vi "releaseQueue.vi"(8 "Error In":errorcluster, 11 "MissionQueue.lvclass":refnum<class "MissionQueue.lvclass">) -> (0 "Error Out":errorcluster, 2 "remaining elements":refnum<class "Mission.lvclass">[](array[class]))   [LabVIEW 2011, in "MissionQueue.lvclass"]
doc: "Close the MissionQueue reference and returning all items remaining in the queue. Note that because this wire works by reference rather than by value, this will close all references in memory to the given MissionQueue.\n\nAuthor: Jared Kirschner"
uses:
  MissionQueue.lvclass
  Mission/Mission.lvclass
  MissionQueue.lvclass/MissionQueue.ctl
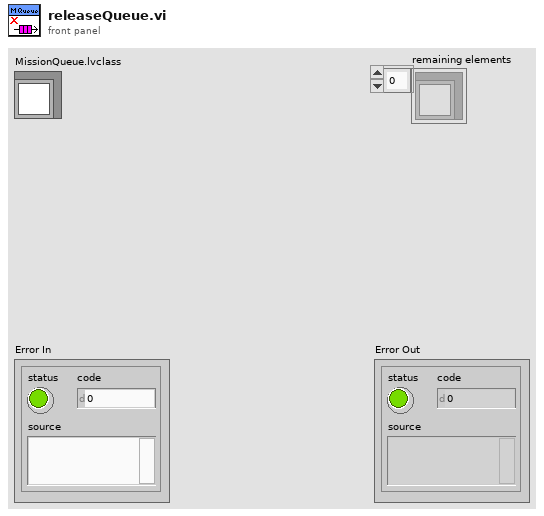
[diagram p1: front panel]
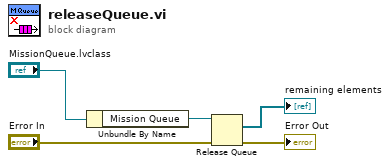
[diagram p0: block diagram]
diagram:
  n1 = Unbundle By Name("MissionQueue.lvclass") -> ("Mission Queue"=w4:refnum<queue>)
  n2 = Release Queue(queue=w4, error in (no error)="Error In") -> (remaining elements=→"remaining elements":refnum<class "Mission.lvclass">[], error out=→"Error Out":errorcluster)  [unwired: 1 in, 1 out]
